vi "okCFrontPanelDevices Constructor.vi"(8 "Error In":errorcluster) -> (0 "Error Out":errorcluster, 2 "okCFrontPanel Refnum":refnum<k24>, 3 "okCFrontPanelDevices Refnum":refnum<k24>)   [LabVIEW 2021, in "okFrontPanelC#Wrapper.lvlib"]
uses:
  okFrontPanelC#Wrapper.lvlib
  D:/UCLA Thinkpad Google Drive/LabVIEW 2021 SP1/builds/SwissSPAD Live Distribution/Opal Kelly/C# Wrapper/v5.0.2/libFrontPanel-csharp.dll
  v5.0.2/libFrontPanel-csharp.dll
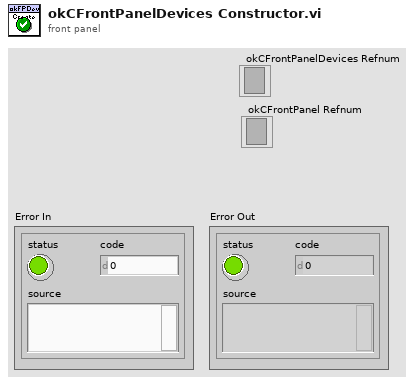
[diagram p1: front panel]
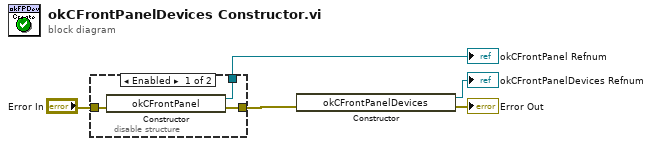
[diagram p0: block diagram]
diagram:
  n1 = disable-structure shown="Enabled" {
    disable-tunnel: "Error In" -> [w8 w9]
    disable-tunnel: [w7 w9] -> w2
    disable-tunnel: [w6 _] -> w1
    frame Enabled {
      n2 = constructor class="okCFrontPanel"(error in=w8) -> (reference out=w6:refnum<k24>, error out=w7:errorcluster)  [unwired: 2 in, 1 out]
    }
    frame Disabled {
    }
  }
  "okCFrontPanel Refnum" <- w1
  n3 = constructor class="okCFrontPanelDevices"(error in=w2) -> (reference out=→"okCFrontPanelDevices Refnum":refnum<k24>, error out=→"Error Out":errorcluster)  [unwired: 2 in, 1 out]
